vi "Create Consumer Queues.vi"() -> (0 "error out":errorcluster, 2 "Consumer Queues":T1)   [LabVIEW 2019, in "TS Framework.lvlib"]
uses:
  TS Framework.lvlib
  Consumer Queues.ctl
  UI Process/Generic UI Command/Generic UI Process Command.lvclass
  DAC Process/Generic DAC Command/Generic DAC Process Command.lvclass
  Trig Process/Generic Trig Command/Generic Trig Process Command.lvclass
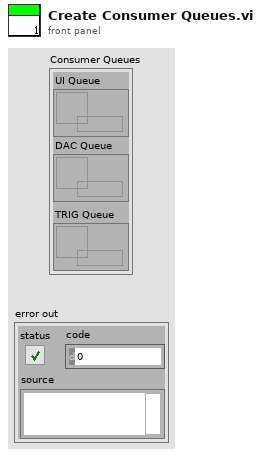
[diagram p1: front panel]
types:
  T1 = typedef "TS Framework.lvlib/Consumer Queues.ctl" = cluster{"UI Queue":refnum<queue>, "DAC Queue":refnum<queue>, "TRIG Queue":refnum<queue>}
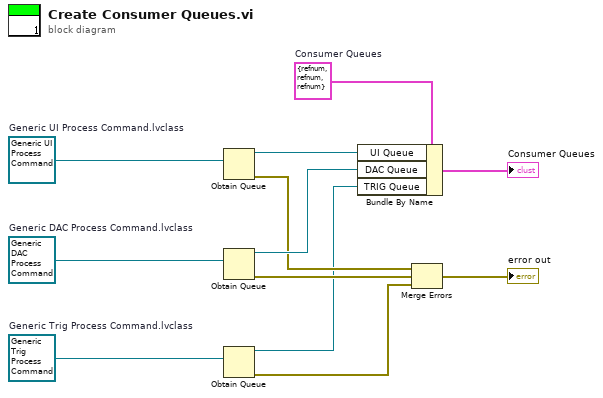
[diagram p0: block diagram]
diagram:
  w3 = refnum<class "Generic Trig Process Command.lvclass"> refnum  # Generic Trig Process Command.lvclass
  w10 = refnum<class "Generic DAC Process Command.lvclass"> refnum  # Generic DAC Process Command.lvclass
  w11 = refnum<class "Generic UI Process Command.lvclass"> refnum  # Generic UI Process Command.lvclass
  w12 = T1 {"UI Queue"=refnum, "DAC Queue"=refnum, "TRIG Queue"=refnum}  # Consumer Queues
  n1 = Obtain Queue(element data type=w11) -> (queue out=w9:refnum<queue>, error out=w5:errorcluster)  [unwired: 4 in, 1 out]
  n2 = Obtain Queue(element data type=w10) -> (queue out=w8:refnum<queue>, error out=w6:errorcluster)  [unwired: 4 in, 1 out]
  n3 = Obtain Queue(element data type=w3) -> (queue out=w2:refnum<queue>, error out=w1:errorcluster)  [unwired: 4 in, 1 out]
  n4 = Bundle By Name(cluster=w12, "UI Queue"=w9, "DAC Queue"=w8, "TRIG Queue"=w2) -> (→"Consumer Queues":T1)
  n5 = Merge Errors(w5, w6, w1) -> (→"error out":errorcluster)
